vi "Close Log File.vi"(8 "error in":errorcluster, 9 "# Rows":u32, 10 "Offset # Rows":u64, 11 "Byte Stream File in":refnum<file>) -> (0 "Error Out":errorcluster, 3 "Byte Stream File out":refnum<file>)   [LabVIEW 2021]
doc: "Author: Scott Hannahs <sth@magnet.fsu.edu>\nCopyright 2018 Florida State University, All rights reserved."
uses:
  RT Host Globals.vi
  <vilib>/regexp/Match Regular Expression.xnode
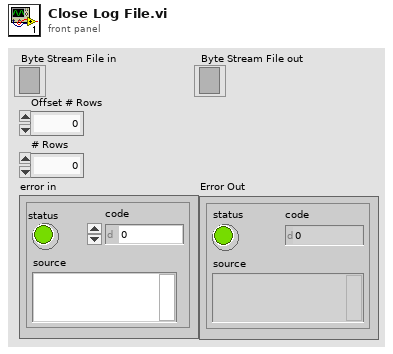
[diagram p1: front panel]
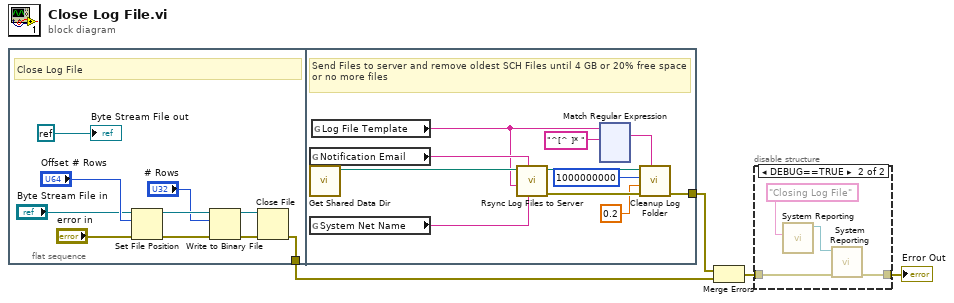
[diagram p0: block diagram]
diagram:
  n1 = flat-sequence {
    tunnel: [w14] -> w4
    tunnel: [w22] -> w3
    frame #0 {
      # "Close Log File"
      n2 = Set File Position(offset (in bytes) (0)="Offset # Rows", refnum="Byte Stream File in", error in="error in") -> (refnum out=w9:refnum<file>, error out=w10:errorcluster)  [unwired: 1 in]
      n3 = Write to Binary File(file (use dialog)=w9, data="# Rows", error in=w10) -> (refnum out=w6:refnum<file>, error out=w5:errorcluster)  [unwired: 3 in, 1 out]
      n4 = Close File(refnum=w6, error in=w5) -> (error out=w14:errorcluster)  [unwired: 1 out]
      "Byte Stream File out" <- refnum<k0> refnum
    }
    frame #1 {
      # "Send Files to server and remove oldest SCH Files until 4 GB or 20% free space or no more files"
      n5 = global read "RT Host Globals.vi" "Notification Email"() -> (w20:string)
      n6 = call "Get Shared Data Dir.vi"() -> ("Data Directory Path"=w21:path)  [unwired: 2 in, 1 out]
      n7 = global read "RT Host Globals.vi" "System Net Name"() -> (w19:string)
      n8 = global read "RT Host Globals.vi" "Log File Template"() -> (w15:string)
      n9 = call "Rsync Log Files to Server.vi"("System Net Name"=w19, "Recipients"=w20, "Log File Template"=w15, "Log File Path In"=w21) -> ("Error Out"=w23:errorcluster, "Log File Path Out"=w25:path)  [unwired: 3 in, 3 out]
      n10 = xnode "Match Regular Expression"("input string"=w15, "regular expression"="^[^ ]* ") -> ("whole match"=w16:string)  [unwired: 4 in, 4 out]
      n11 = call "Cleanup Log Folder.vi"("Template"=w16, "Error In"=w23, "Min Fraction"=0.2, "Min Space"=i64 1000000000 ("y"), "Log File Path In"=w25) -> ("Error Out"=w22:errorcluster)  [unwired: 6 in]
    }
  }
  n12 = Merge Errors(w3, w4) -> (w2:errorcluster)
  n13 = disable-structure shown="DEBUG==TRUE" {
    disable-tunnel: w2 -> [w143 w145]
    disable-tunnel: [w143 w144] -> w1
    frame condition #0 (active) {
    }
    frame condition #1 {
      n14 = call "System Reporting.vi"("String"="Closing Log File") -> ("Byte Stream File out"=w147:refnum<file>)  [unwired: 9 in, 1 out]
      n15 = call "System Reporting.vi"("Error In"=w145, "Byte Stream File in"=w147) -> ("Error Out"=w144:errorcluster)  [unwired: 8 in, 1 out]
    }
  }
  "Error Out" <- w1
